vi "Write AnalysisConfig.vi"(8 "error in (no error)":errorcluster, 10 "clAnalysisConfig":T1={"F0"=60, "SettlingTime"=7.0, "AnalysisCycles"=20.0, "SampleRate"=4800.0, "NumChannels"=6, "TsOffset"=enum."start"}, 11 "Fitter in":refnum<class "FitterBase.lvclass">) -> (0 "error out":errorcluster, 3 "Fitter out":refnum<class "FitterBase.lvclass">)   [LabVIEW 2014, in "AnalysisPlugins.lvlib" / "FitterBase.lvclass"]
uses:
  FitterBase.lvclass
  Typedefs/clAnalysisConfig.ctl
  FitterBase.lvclass/FitterBase.ctl
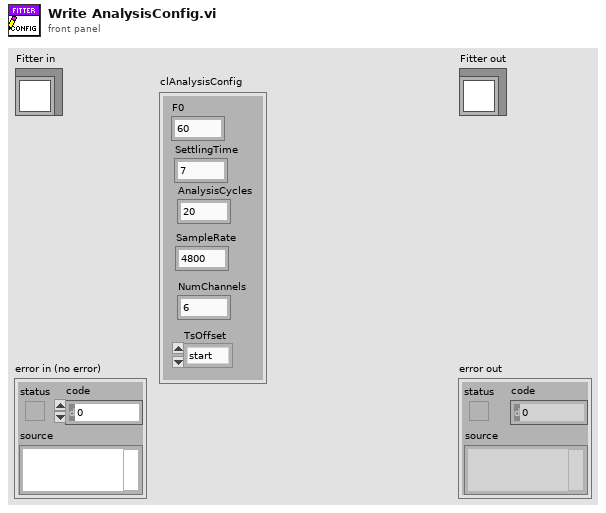
[diagram p1: front panel]
types:
  T1 = typedef "AnalysisPlugins.lvlib/FitterBase.lvclass/clAnalysisConfig.ctl" = cluster{"F0":u32, "SettlingTime":dbl, "AnalysisCycles":dbl, "SampleRate":dbl, "NumChannels":u32, "TsOffset":enum16{"start", "middle", "end"}}
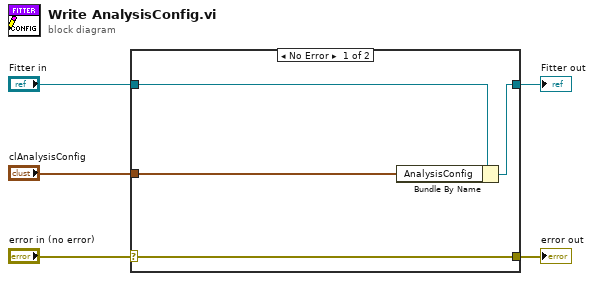
[diagram p0: block diagram]
diagram:
  n1 = case shown="No Error" "error in (no error)" {
    selector: "error in (no error)" -> [w9 w10]
    tunnel: [w9 w10] -> w4
    tunnel: [w7 w11] -> w2
    tunnel: "Fitter in" -> [w8 w11]
    tunnel: "clAnalysisConfig" -> [w6 _]
    frame No Error {
      n2 = Bundle By Name(cluster=w8, "AnalysisConfig"=w6) -> (w7:refnum<class "FitterBase.lvclass">)
    }
    frame Error {
    }
  }
  "error out" <- w4
  "Fitter out" <- w2
